vi "Terminal-Global-ReferenceValues.vi"() -> ()   [LabVIEW 2014]
panel:
  in  "性能监测子系统测控参数":T1
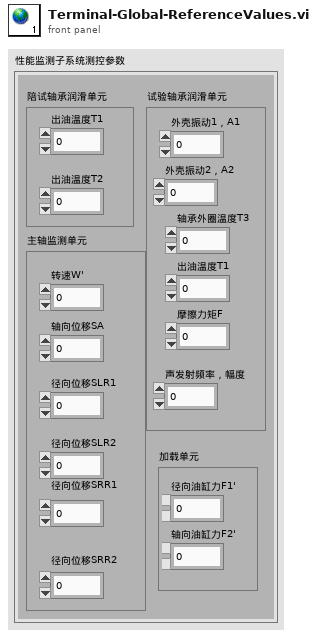
[diagram p1: front panel]
types:
  T1 = cluster{"陪试轴承润滑单元":cluster{"出油温度T1":dbl, "出油温度T2":dbl}, "试验轴承润滑单元":cluster{"外壳振动1，A1":dbl, "外壳振动2，A2":dbl, "轴承外圈温度T3":dbl, "出油温度T1":dbl, "摩擦力矩F":dbl, "声发射频率，幅度":dbl}, "加载单元":cluster{"径向油缸力F1'":dbl, "轴向油缸力F2'":dbl}, "主轴监测单元":cluster{"转速W'":dbl, "轴向位移SA":dbl, "径向位移SLR1":dbl, "径向位移SLR2":dbl, "径向位移SRR1":dbl, "径向位移SRR2":dbl}}
diagram:
